vi "Vision Processing.vi"(4 "error in (no error)":errorcluster) -> ()   [LabVIEW 2013]
doc: "This VI runs in parallel to other tasks. It gets images from the camera, processes them for color or shape and use that information to affect robot behavior."
uses:
  <vilib>/Rock Robotics/WPI/Camera/WPI_CameraWhite Balance Values.ctl
  <vilib>/Rock Robotics/WPI/Camera/WPI_CameraExposure Values.ctl
  <vilib>/Rock Robotics/WPI/Camera/WPI_CameraFrameRate.ctl
  <vilib>/Rock Robotics/WPI/Camera/WPI_CameraImageSize.ctl
  <vilib>/Rock Robotics/WPI/Camera/WPI_CameraSettings Read MJPG.ctl
  Robot Global Data.vi
panel:
  out "Error":bool
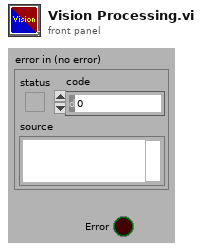
[diagram p1: front panel]
types:
  T1 = typedef "WPI_CameraImageSize.ctl" = enum16{"640x480", "320x240", "160x120"}
  T2 = typedef "WPI_CameraFrameRate.ctl" = u32
  T3 = typedef "WPI_CameraExposure Values.ctl" = enum16{"Auto", "Flicker-free 50 Hz", "Flicker-free 60 Hz", "Hold current"}
  T4 = typedef "WPI_CameraWhite Balance Values.ctl" = enum16{"Auto", "Fixed indoor", "Fixed outdoor 1", "Fixed outdoor 2", "Fixed fluorescent 1", "Fixed fluorescent 2", "Hold current"}
  T5 = typedef "Image Type" = u32
  T6 = typedef "WPI_CameraDevRef.ctl" = cluster{"Camera Address":string, "CameraStatus":errorcluster, "Acquire Image Notifier":refnum<notifier>}
  T7 = typedef "IMAQ Image.ctl" = refnum<image>
  T8 = cluster{"Hue":cluster{dbl, dbl}, "Sat":cluster{dbl, dbl}, "Val":cluster{dbl, dbl}}
  T9 = typedef "WPI_CameraSettings Read MJPG.ctl" = cluster{"fps":i32, "compression":i32, "Image Size":T1}
  T10 = cluster{"Horizontal":bool, "Aspect Score":dbl, "Rect Score":dbl, cluster{"Left":dbl, "Top":dbl, "Right":dbl, "Bottom":dbl}, "Equiv H":dbl, "Equiv V":dbl}[]
  T11 = cluster{cluster{dbl, dbl}, cluster{dbl, dbl}, cluster{dbl, dbl}}
  T12 = typedef "TargetType.ctl" = enum16{"Not Hot", "Hot"}
  T13 = cluster{"Scores":cluster{"Total":dbl, "Left":dbl, "Right":dbl, "Ratio":dbl, "Vertical":dbl, "index":i32, "State":T12}, "Verticals":cluster{"Horizontal?":bool, "Aspect Score":dbl, "Rect Score":dbl, cluster{"Left":dbl, "Top":dbl, "Right":dbl, "Bottom":dbl}, "Equiv H":dbl, "Equiv V":dbl}, "Horizontals":cluster{"Horizontal?":bool, "Aspect Score":dbl, "Rect Score":dbl, cluster{"Left":dbl, "Top":dbl, "Right":dbl, "Bottom":dbl}, "Equiv H":dbl, "Equiv V":dbl}, "Validated":bool}[]
  T14 = cluster{"Scores":cluster{"Total":dbl, "Left":dbl, "Right":dbl, "Ratio":dbl, "Vertical":dbl, "index":i32, "State":T12}, "Verticals":cluster{"Horizontal?":bool, "Aspect Score":dbl, "Rect Score":dbl, cluster{"Left":dbl, "Top":dbl, "Right":dbl, "Bottom":dbl}, "Equiv H":dbl, "Equiv V":dbl}, "Horizontals":cluster{"Horizontal?":bool, "Aspect Score":dbl, "Rect Score":dbl, cluster{"Left":dbl, "Top":dbl, "Right":dbl, "Bottom":dbl}, "Equiv H":dbl, "Equiv V":dbl}, "Distance (ft)":dbl, "Target Center (-1 to 1)":cluster{"X":dbl, "Y":dbl}}[]
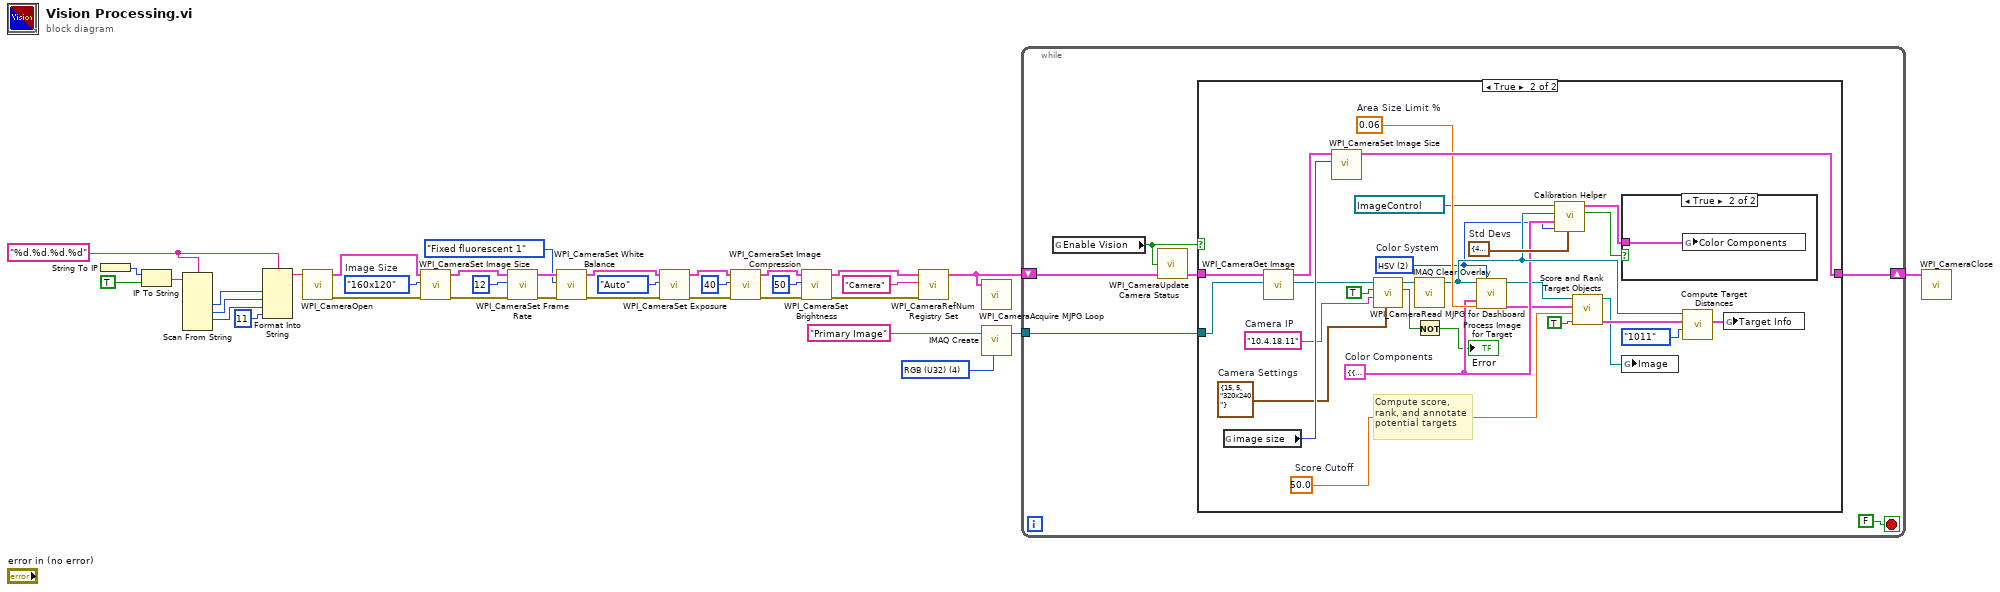
[diagram p0: block diagram]
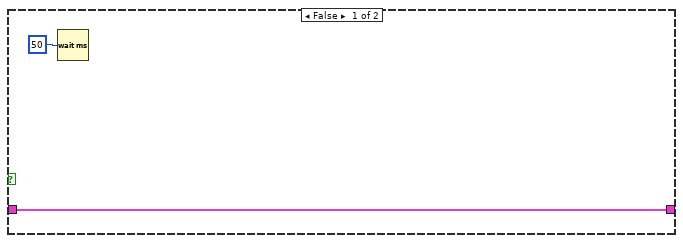
[diagram p2: hidden frame]
diagram:
  w1 = WPI_CameraImageSize."160x120"  # Image Size
  w5 = "%d.%d.%d.%d" ("format string")
  w35 = T5 4 items=["Grayscale (U8)", "Grayscale (I16)", "Grayscale (SGL)", "Complex (CSG)", "RGB (U32)", "HSL (U32)", "RGB (U64)"] ("Image Type")
  n1 = String To IP() -> (0:w12:u32)  [unwired: 1 in]
  n2 = IP To String(1:TRUE ("dot notation? (F)"), 2:w12) -> (0:w10:string)
  n3 = Scan From String(format string=w5, input string=w10) -> (output 1=w9:i32, output 2=w8:i32, output 3=w7:i32)  [unwired: 7 in, 3 out]
  n4 = Format Into String(format string=w5, w9, w8, w7, 11 ("Compression")) -> (resulting string=w4:string)  [unwired: 2 in, 1 out]
  n5 = call <vilib>:"WPI_CameraOpen.vi"("Camera Address"=w4) -> ("error out"=w23:errorcluster, "CameraDevRef"=w24:T6)  [unwired: 1 in, 8 out]
  n6 = call <vilib>:"WPI_CameraSet Image Size.vi"("error in (no error)"=w23, "Image Size"=w1, "CameraDevRef"=w24) -> ("error out"=w22:errorcluster, "CameraDevRef Out"=w25:T6)  [unwired: 7 out]
  n7 = call <vilib>:"WPI_CameraSet Frame Rate.vi"("error in (no error)"=w22, "Frame Rate (fps)"=T2 12, "CameraDevRef"=w25) -> ("error out"=w21:errorcluster, "CameraDevRef Out"=w27:T6)  [unwired: 7 out]
  n8 = call <vilib>:"WPI_CameraSet White Balance.vi"("error in (no error)"=w21, "White Balance"=WPI_CameraWhite_Balance_Values."Fixed fluorescent 1", "CameraDevRef"=w27) -> ("error out"=w20:errorcluster, "CameraDevRef Out"=w26:T6)  [unwired: 7 out]
  n9 = call <vilib>:"WPI_CameraSet Exposure.vi"("error in (no error)"=w20, "Exposure"=WPI_CameraExposure_Values."Auto", "CameraDevRef"=w26) -> ("error out"=w19:errorcluster, "CameraDevRef Out"=w29:T6)  [unwired: 7 out]
  n10 = call <vilib>:"WPI_CameraSet Image Compression.vi"("error in (no error)"=w19, "Compression"=40, "CameraDevRef"=w29) -> ("error out"=w18:errorcluster, "CameraDevRef Out"=w28:T6)  [unwired: 7 out]
  n11 = call <vilib>:"WPI_CameraSet Brightness.vi"("error in (no error)"=w18, "Brightness"=50, "CameraDevRef"=w28) -> ("error out"=w16:errorcluster, "CameraDevRef Out"=w17:T6)  [unwired: 7 out]
  n12 = call <vilib>:"WPI_CameraRefNum Registry Set.vi"("error in (no error)"=w16, "refnum name"="Camera", "CameraDevRef"=w17) -> ("CameraDevRef"=w3:T6)  [unwired: 8 out]
  n13 = call <vilib>:"WPI_CameraAcquire MJPG Loop.vi"("CameraDevRef"=w3) -> ()  [unwired: 11 in]
  n14 = call "IMAQ Create"("Image Name"="Primary Image", "Image Type"=w35) -> ("New Image"=w33:T7)  [unwired: 2 in, 2 out]
  n15 = while {
    shift-right: [w40] -> w2
    shift-left: w3 -> [w38]
    tunnel: w33 -> [w39]
    stop <- FALSE stop-if-true
    n16 = global read "Robot Global Data.vi" "Enable Vision"() -> (w36:bool)
    n17 = call <vilib>:"WPI_CameraUpdate Camera Status.vi"("CameraDevRef In"=w38, "Enable Vision"=w36) -> ("CameraDevRef Out"=w37:T6)  [unwired: 3 in]
    n18 = case shown="True" w36 {
      tunnel: w39 -> [_ w70]
      tunnel: [w43 w71] -> w40
      tunnel: w37 -> [w43 w68]
      frame False {
        n19 = Wait (ms)(milliseconds to wait=u32 50) -> ()  [unwired: 1 out]
      }
      frame True {
        w55 = T8 {"Hue"={80.65384674072266, 112.65384674072266}, "Sat"={49.712730407714844, 255.0}, "Val"={73.74692153930664, 173.4838523864746}}  # Color Components
        w66 = cluster{"Hue":dbl, "Sat":dbl, "Val":dbl} {"Hue"=4.0, "Sat"=6.0, "Val"=4.0}  # Std Devs
        w65 = 50.0  # Score Cutoff
        w64 = 0.06  # Area Size Limit %
        w63 = T9 {"fps"=15, "compression"=5, "Image Size"=enum."320x240"}  # Camera Settings
        w62 = "10.4.18.11"  # Camera IP
        w53 = u16 2 items=["RGB", "HSL", "HSV", "HSI"]  # Color System
        # "Compute score,\nrank, and annotate\npotential targets"
        n20 = global read "Robot Global Data.vi" "image size"() -> (w69:T1)
        n21 = call <vilib>:"WPI_CameraGet Image.vi"("Image"=w70, "CameraDevRef"=w68) -> ("Image Out"=w47:T7, "CameraDevRef Out"=w67:T6)  [unwired: 1 in, 7 out]
        n22 = call <vilib>:"WPI_CameraSet Image Size.vi"("Image Size"=w69, "CameraDevRef"=w67) -> ("CameraDevRef Out"=w71:T6)  [unwired: 1 in, 8 out]
        n23 = call <vilib>:"WPI_CameraRead MJPG for Dashboard.vi"("Camera Settings"=w63, "Camera IP"=w62, "Enable"=TRUE, "Refnum in"=w47) -> ("Active"=w60:bool, "Refnum out"=w48:T7)  [unwired: 4 in, 2 out]
        n24 = call "IMAQ Clear Overlay"("Image"=w48) -> ("Image Out"=w57:T7)  [unwired: 9 in, 1 out]
        n25 = Not(x=w60) -> (.not. x?=→"Error":bool)
        n26 = call "Process Image for Target.vi"("Src Image"=w57, "Color Mode"=w53, "Color Components"=w55, "Area Cutoff %"=w64) -> ("Src Image Out"=w50:T7, "Particles"=w51:T10)  [unwired: 9 in, 1 out]
        n27 = call "Calibration Helper.vi"("Std Devs"=w66, "Color Mode"=w53, "Color Components"=w55, "Image"=w57, "Image Ctl Refnum"=refnum<vi> refnum ("Image")) -> ("Changed"=w56:bool, "output color"=w54:T11)  [unwired: 5 in]
        n28 = call "Score and Rank Target Objects.vi"("Annotate"=TRUE, "Score Limit"=w65, "Particles"=w51, "Image in"=w50) -> ("Target Info"=w52:T13, "Annotated Image"=w45:T7)  [unwired: 6 in]
        n29 = case shown="True" w56 {
          tunnel: w54 -> [_ w72]
          frame False {
          }
          frame True {
            n30 = global write "Robot Global Data.vi" "Color Components"(w72) -> ()
          }
        }
        n31 = global write "Robot Global Data.vi" "Image"(w45) -> ()
        n32 = call "Compute Target Distances.vi"("Camera Type"=enum16{"206", "1011", "1013"}."1011", "Target Info"=w52, "Image in"=w57) -> ("Target Info"=w46:T14)  [unwired: 6 in, 2 out]
        n33 = global write "Robot Global Data.vi" "Target Info"(w46) -> ()
      }
    }
  }
  n34 = call <vilib>:"WPI_CameraClose.vi"("CameraDevRef"=w2) -> ()  [unwired: 1 in, 10 out]
